vi "c_ctre_phoenix6_RequestControlDiff_TorqueCurrentFOC_Velocity.vi"(0 "String 2":string, 1 "Numeric 2":u32, 2 "Numeric 3":dbl, 3 "Numeric 4":dbl, 4 "Numeric 5":dbl, 5 "Numeric 6":dbl, 6 "Numeric 7":u8, 7 "Numeric 8":u8, 8 "Numeric 9":u8, 9 "Numeric 10":u8, 10 "Numeric 11":u8, 11 "Numeric 12":dbl, 12 "Numeric 13":dbl, 13 "Numeric 14":dbl, 14 "Numeric 15":i32, 15 "Numeric 16":u8, 16 "Numeric 17":u8, 17 "Numeric 18":u8, 18 "Numeric 19":u8, 19 "Numeric 20":u8) -> (20 "Numeric":i32, 21 "String":string)   [LabVIEW 2023]
uses:
  <vilib>/Rock Robotics/WPI/ThirdParty/Phoenix-LabVIEW/Controls/DriverLib.ctl
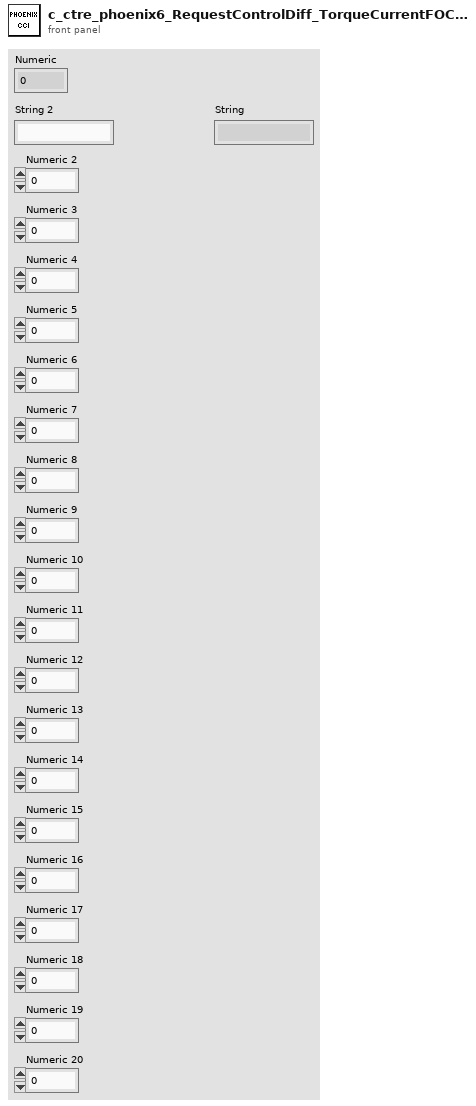
[diagram p1: front panel]
types:
  T1 = typedef "DriverLib.ctl" = path
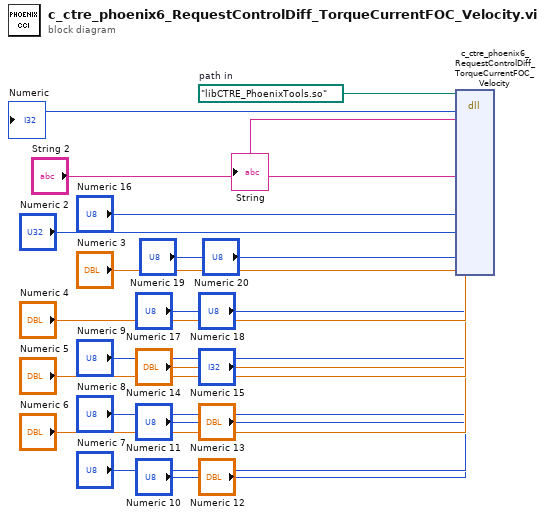
[diagram p0: block diagram]
diagram:
  w23 = T1 path "libCTRE_PhoenixTools.so"  # path in
  n1 = dll-call lib="?" fn="c_ctre_phoenix6_RequestControlDiff_TorqueCurrentFOC_Velocity"(path in=w23, "String 2", "Numeric 2", "Numeric 3", "Numeric 4", "Numeric 5", "Numeric 6", "Numeric 7", "Numeric 8", "Numeric 9", "Numeric 10", "Numeric 11", "Numeric 12", "Numeric 13", "Numeric 14", "Numeric 15", "Numeric 16", "Numeric 17", "Numeric 18", "Numeric 19", "Numeric 20") -> (→"Numeric":i32, →"String":string)  [unwired: 21 in, 2 out]
